vi "UIMessage1.vi"(4 "User Parameter":T1, 5 "Event Data":cluster{"uiMsg":refnum<k7>, "cancel":bool}, 6 "Control Ref":refnum<k7>, 7 "Event Common Data":T2) -> (1 "Event Data Out":cluster{"cancel":bool})   [LabVIEW 2018]
uses:
  <vilib>/Utility/miscctls.llb/LVRowAndColumnUnsignedTypeDef.ctl
  <vilib>/Utility/miscctls.llb/LVRowAndColumnTypeDef.ctl
  <vilib>/Utility/file.llb/Write Delimited Spreadsheet (string).vi
panel:
  in  "error in (no error)":errorcluster
  out "reference out":refnum<vi>
  out "error out":errorcluster
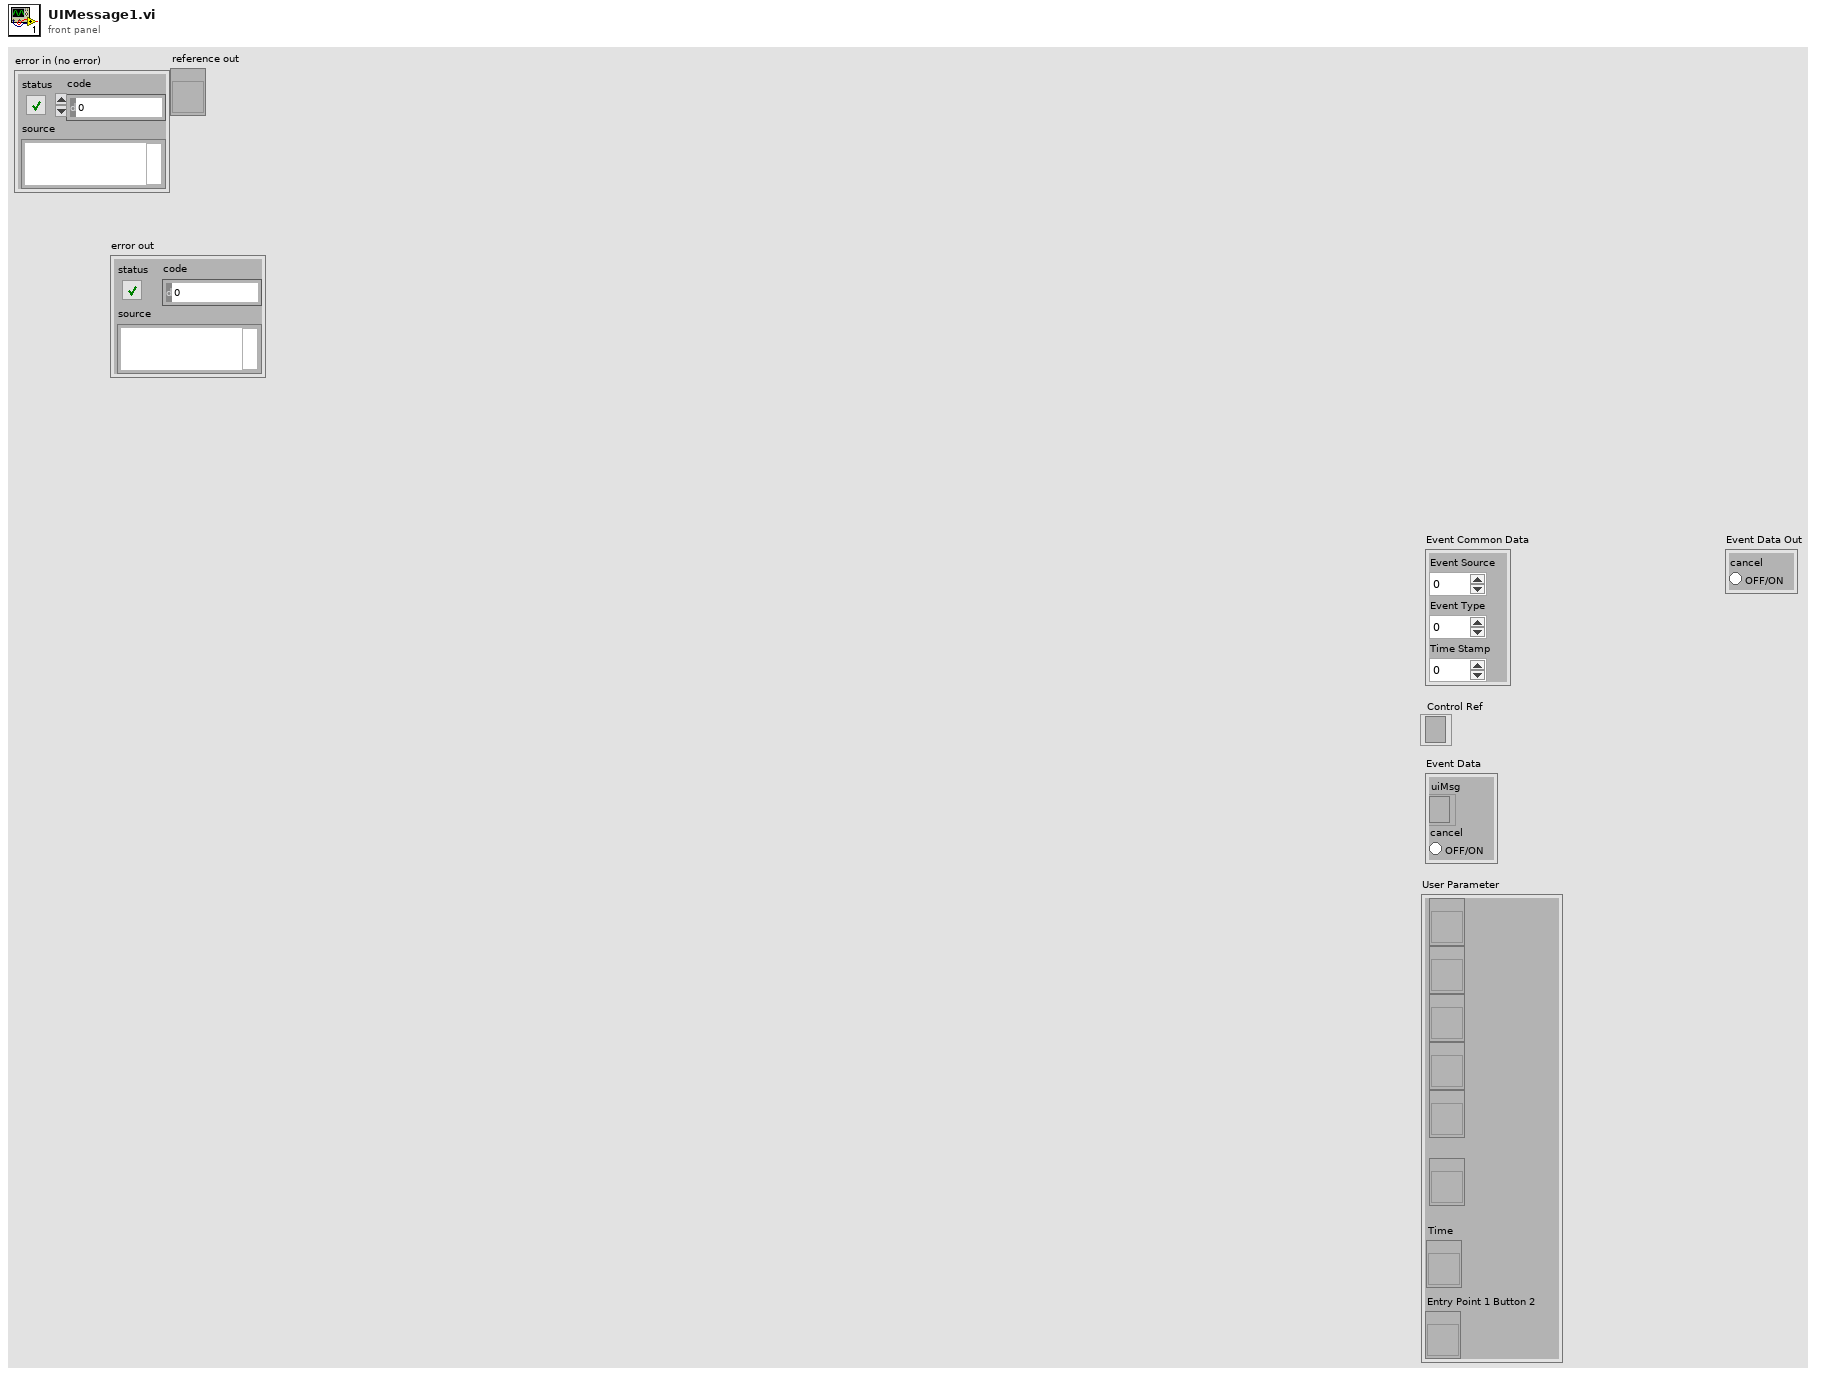
[diagram p1: front panel]
types:
  T1 = cluster{refnum<vi>, refnum<vi>, refnum<vi>, refnum<vi>, refnum<vi>, refnum<vi>, "Time":refnum<vi>, "Entry Point 1 Button 2":refnum<vi>}
  T2 = cluster{"Event Source":i32, "Event Type":u32, "Time Stamp":u32}
  T3 = typedef "LVRowAndColumnUnsignedTypeDef.ctl" = cluster{"Row":u32, "Column":u32}
  T4 = enum8{"Enabled", "Disabled", "Disabled and Grayed Out"}
  T5 = typedef "LVRowAndColumnTypeDef.ctl" = cluster{"Row":i32, "Column":i32}
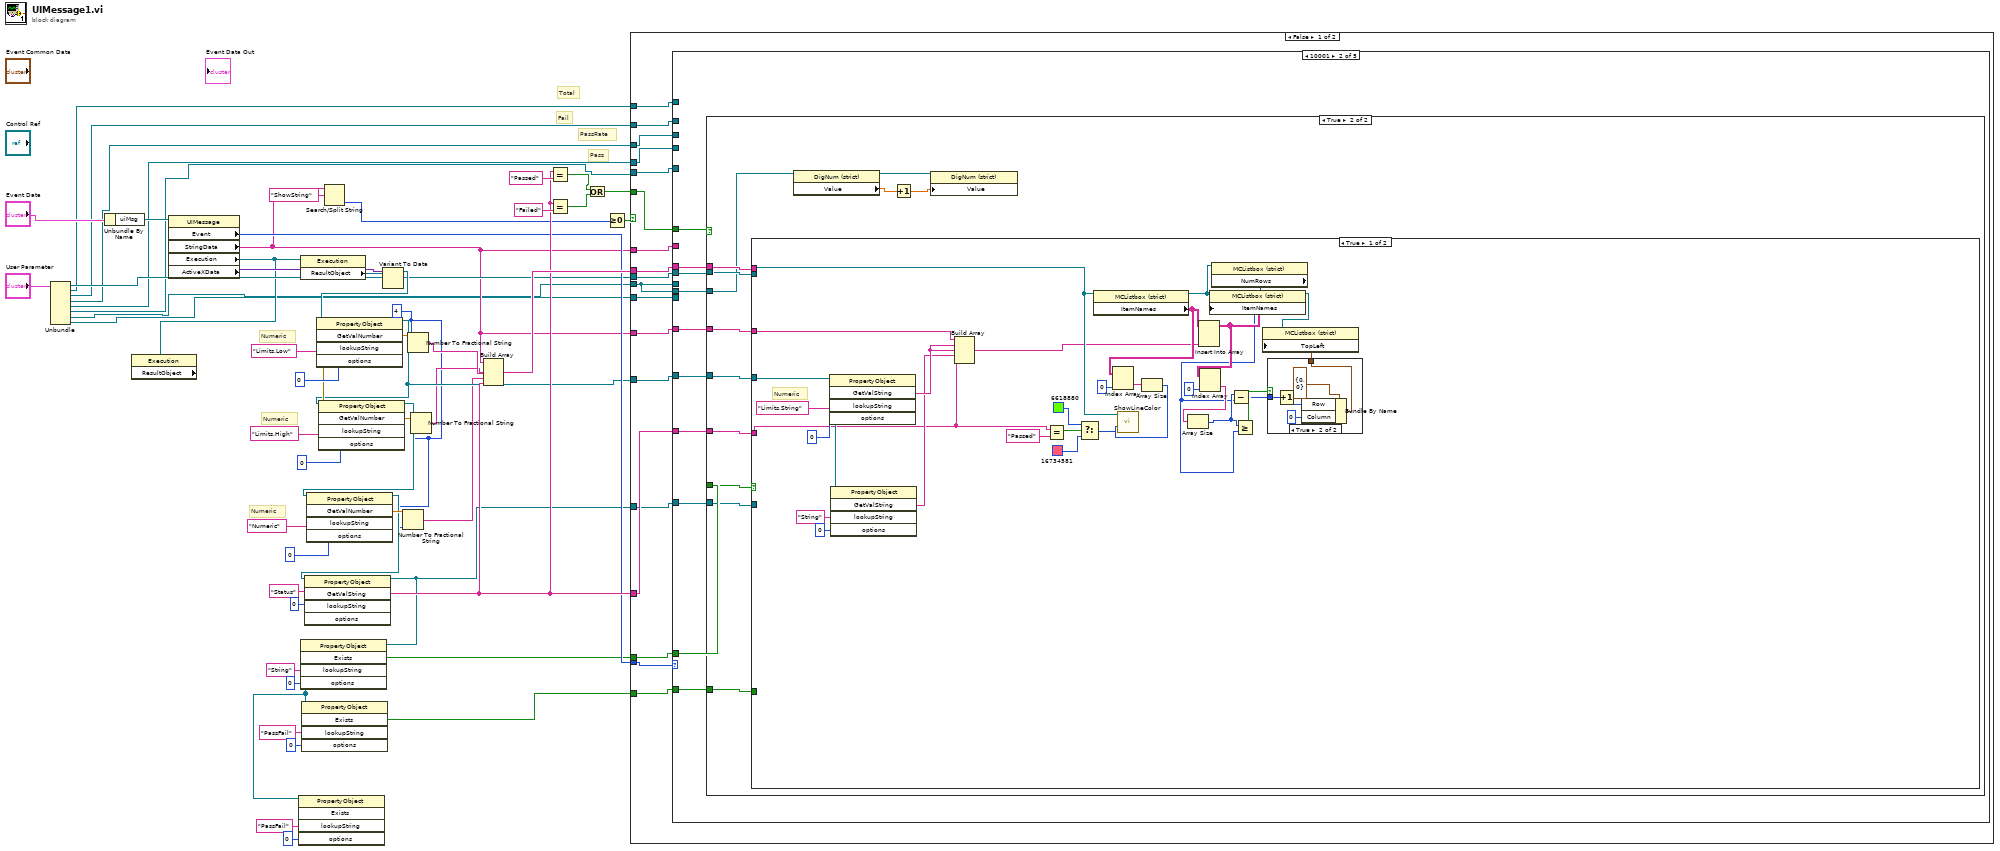
[diagram p0: block diagram]
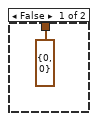
[diagram p4: hidden frame]
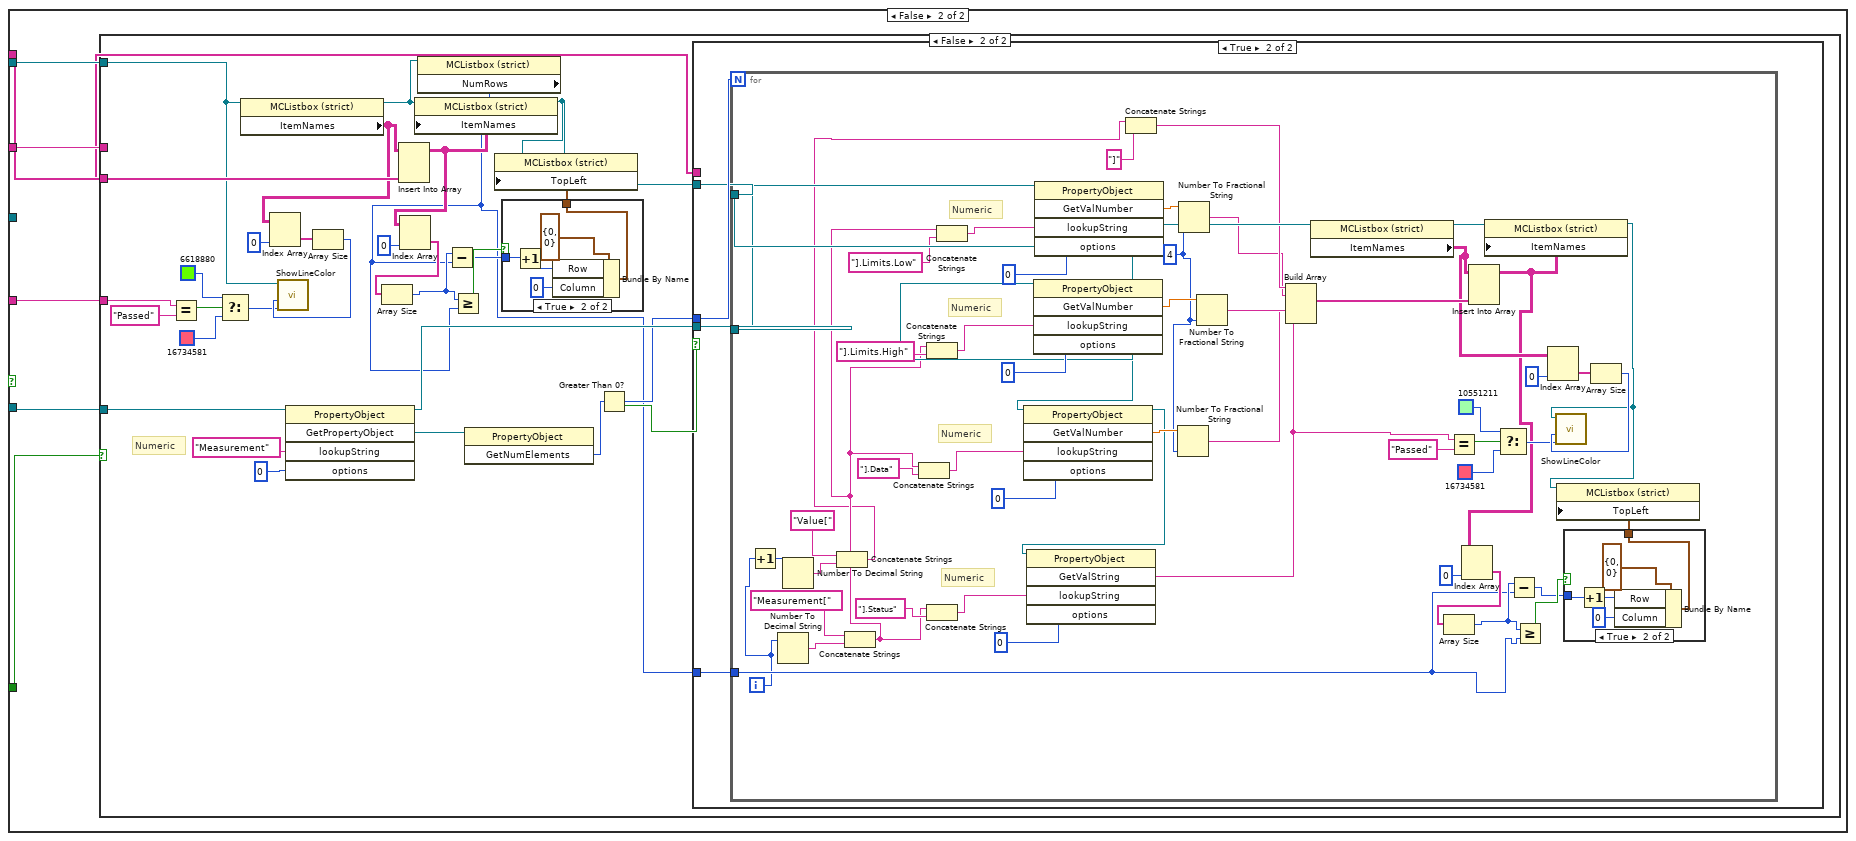
[diagram p5: hidden frame]
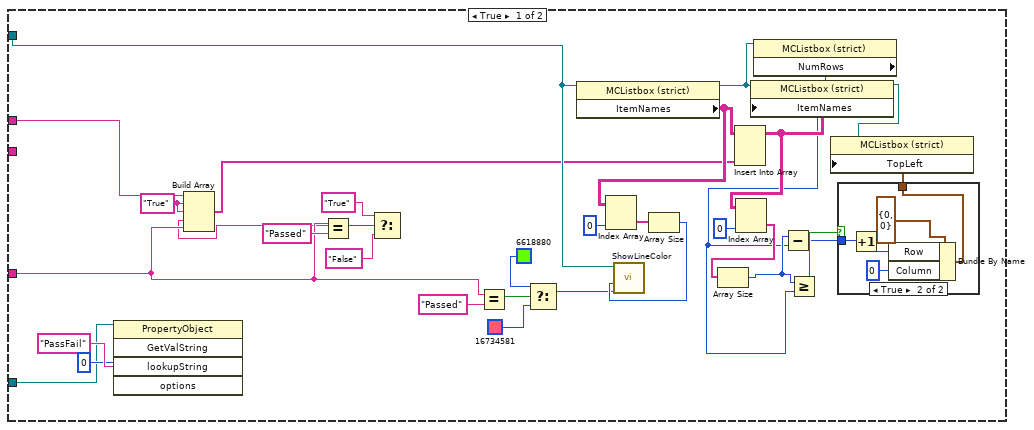
[diagram p6: hidden frame]
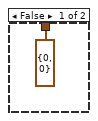
[diagram p7: hidden frame]
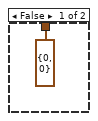
[diagram p8: hidden frame]
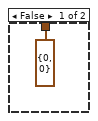
[diagram p10: hidden frame]
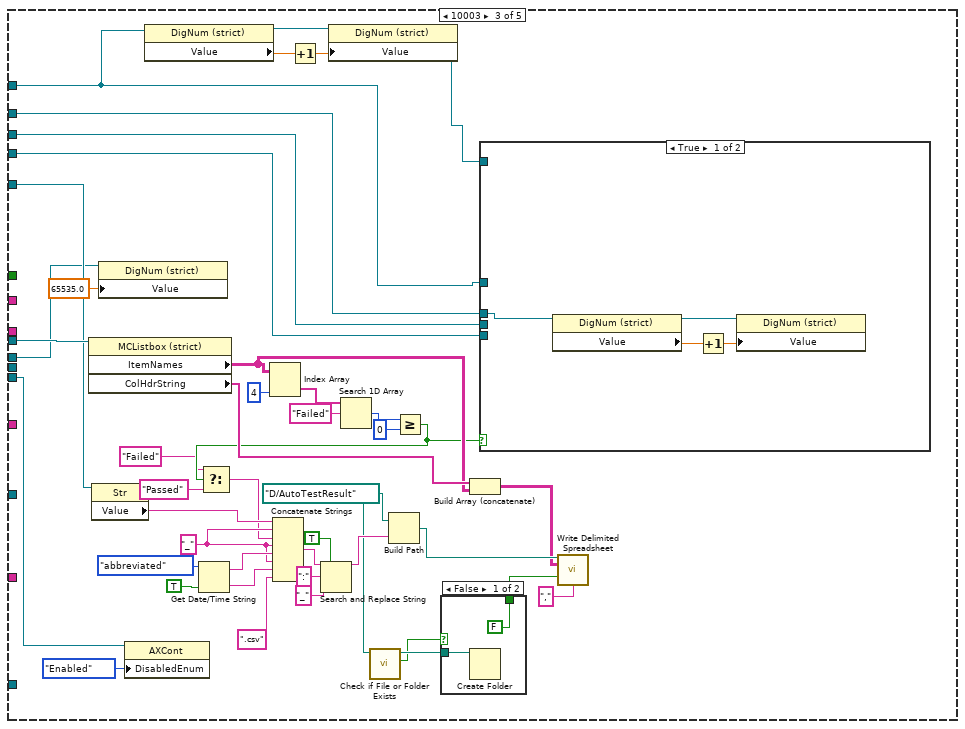
[diagram p11: hidden frame]
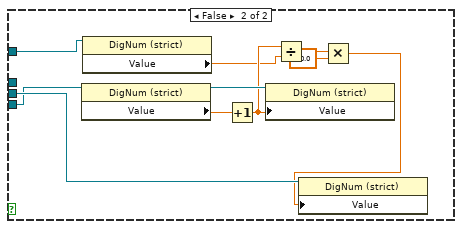
[diagram p13: hidden frame]
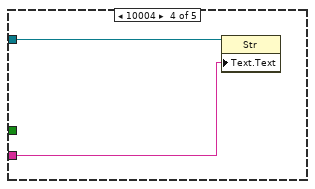
[diagram p14: hidden frame]
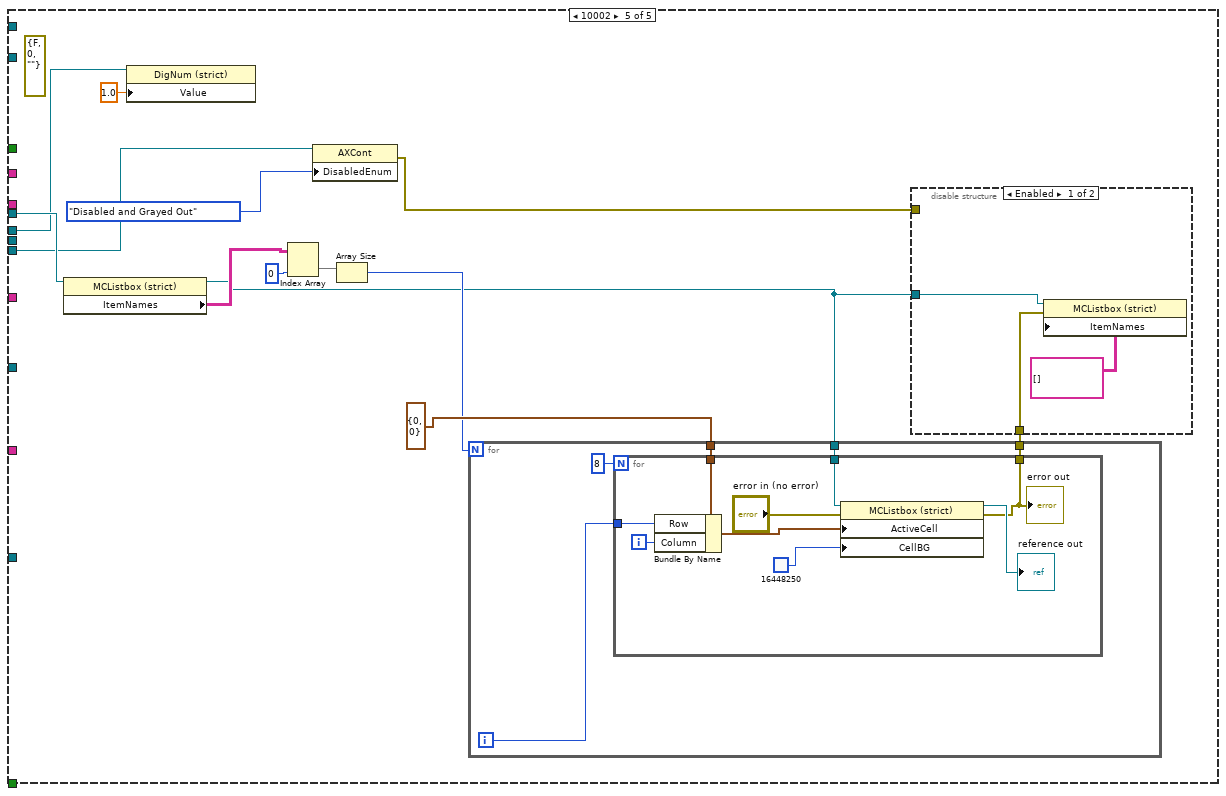
[diagram p15: hidden frame]
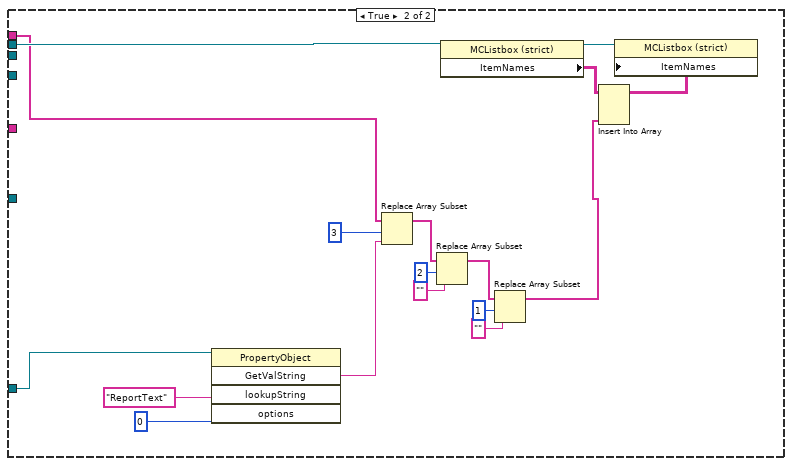
[diagram p17: hidden frame]
diagram:
  w12 = i16 4 ("precision (6)")
  # "Pass"
  # "PassRate"
  # "Fail"
  # "Total"
  # "Numeric"
  # "Numeric"
  # "Numeric"
  n1 = Unbundle("User Parameter") -> (w29:refnum<vi>, w24:refnum<vi>, w27:refnum<vi>, w26:refnum<vi>, w25:refnum<vi>, w4:refnum<vi>, "Time"=w1:refnum<vi>, "Entry Point 1 Button 2"=w2:refnum<vi>)
  n2 = Unbundle By Name("Event Data") -> ("uiMsg"=w56:refnum<k7>)
  n3 = property class="UIMessage"(reference=w56) -> ("Event"=w32:i32, "StringData"=w3:string, "Execution"=w8:refnum<k7>, "ActiveXData"=w55:variant)  [unwired: 1 in, 2 out]
  n4 = property class="Execution" props=["ResultObject"](reference=w8) -> ()  [unwired: 1 in, 3 out]
  n5 = property class="Execution"(reference=w8) -> ("ResultObject"=w52:refnum<k7>)  [unwired: 1 in, 2 out]
  n6 = Search/Split String(string=w3, search string/char (-)="ShowString") -> (offset of match=w6:i32)  [unwired: 1 in, 2 out]
  n7 = Variant To Data(type=w52, Variant=w55) -> (data=w40:refnum<k7>)  [unwired: 1 in, 1 out]
  n8 = invoke class="PropertyObject" method="GetValNumber"(reference=w40, "lookupString"="Limits.Low", "options"=0) -> (reference out=w19:refnum<k7>, error out=w42:errorcluster, "GetValNumber"=w46:dbl)  [unwired: 2 in, 2 out]
  n9 = invoke class="PropertyObject" method="GetValNumber"(reference=w19, error in=w42, "lookupString"="Limits.High", "options"=0) -> (reference out=w39:refnum<k7>, "GetValNumber"=w45:dbl)  [unwired: 1 in, 3 out]
  n10 = invoke class="PropertyObject" method="GetValNumber"(reference=w39, "lookupString"="Numeric", "options"=0) -> (reference out=w38:refnum<k7>, "GetValNumber"=w49:dbl)  [unwired: 2 in, 3 out]
  n11 = invoke class="PropertyObject" method="GetValString"(reference=w38, "lookupString"="Status", "options"=0) -> (reference out=w23:refnum<k7>, "GetValString"=w33:string)  [unwired: 2 in, 3 out]
  n12 = invoke class="PropertyObject" method="Exists"(reference=w23, "lookupString"="String", "options"=0) -> (reference out=w9:refnum<k7>, "Exists"=w20:bool)  [unwired: 2 in, 3 out]
  n13 = invoke class="PropertyObject" method="Exists"(reference=w9, "lookupString"="PassFail", "options"=0) -> ()  [unwired: 2 in, 5 out]
  n14 = invoke class="PropertyObject" method="Exists"(reference=w9, "lookupString"="PassFail", "options"=0) -> ("Exists"=w16:bool)  [unwired: 2 in, 4 out]
  n15 = Number To Fractional String(number=w49, precision (6)=w12) -> (F-format string=w13:string)  [unwired: 2 in]
  n16 = Number To Fractional String(number=w46, precision (6)=w12) -> (F-format string=w15:string)  [unwired: 2 in]
  n17 = Number To Fractional String(number=w45, precision (6)=w12) -> (F-format string=w14:string)  [unwired: 2 in]
  n18 = Build Array(w3, w15, w14, w13, w33) -> (w41:string[])
  n19 = Equal?(x=w33, y="Passed") -> (x = y?=w35:bool)
  n20 = Equal?(x=w33, y="Failed") -> (x = y?=w34:bool)
  n21 = Or(x=w35, y=w34) -> (x .or. y?=w31:bool)
  n22 = Greater Or Equal To 0?(x=w6) -> (x >= 0?=w5:bool)
  n23 = case shown="False" w5 {
    tunnel: w41 -> [w74 w379]
    tunnel: w33 -> [w73 _]
    tunnel: w32 -> [w72 _]
    tunnel: w31 -> [w71 _]
    tunnel: w29 -> [w70 w383]
    tunnel: w27 -> [w69 _]
    tunnel: w26 -> [w68 _]
    tunnel: w25 -> [w67 _]
    tunnel: w24 -> [w66 _]
    tunnel: w23 -> [w65 w380]
    tunnel: w20 -> [w64 _]
    tunnel: w19 -> [w63 _]
    tunnel: w16 -> [w62 _]
    tunnel: w3 -> [w61 _]
    tunnel: w4 -> [w60 _]
    tunnel: w3 -> [w59 _]
    tunnel: w2 -> [w58 _]
    tunnel: w1 -> [w57 _]
    frame False {
      n24 = case shown="10001" w72 {
        tunnel: w74 -> [_ w84 _ _ _]
        tunnel: w70 -> [_ w83 w321 _ w348]
        tunnel: w71 -> [_ w82 _ _ _]
        tunnel: w65 -> [_ w81 _ _ _]
        tunnel: w73 -> [_ w80 _ _ _]
        tunnel: w66 -> [_ _ w310 _ _]
        tunnel: w69 -> [_ _ w315 _ _]
        tunnel: w68 -> [_ _ w313 _ _]
        tunnel: w67 -> [_ _ w314 _ _]
        tunnel: w64 -> [_ w79 _ _ _]
        tunnel: w61 -> [_ w78 _ _ _]
        tunnel: w63 -> [_ w77 _ _ _]
        tunnel: w62 -> [_ w76 _ _ _]
        tunnel: w60 -> [_ _ w307 w339 _]
        tunnel: w59 -> [_ _ _ w338 _]
        tunnel: w58 -> [_ _ w281 _ w344]
        tunnel: w57 -> [_ _ w279 _ w340]
        tunnel: w57 -> [_ w75 _ _ _]
        frame 0, Default {
        }
        frame 10001 {
          n25 = case shown="True" w82 {
            tunnel: w84 -> [_ w96]
            tunnel: w83 -> [_ w94]
            tunnel: w81 -> [_ w95]
            tunnel: w80 -> [_ w93]
            tunnel: w79 -> [_ w92]
            tunnel: w78 -> [_ w91]
            tunnel: w77 -> [_ w90]
            tunnel: w76 -> [_ w89]
            tunnel: w75 -> [_ w86]
            frame False {
            }
            frame True {
              n26 = case shown="True" w92 {
                tunnel: w96 -> [_ w139]
                tunnel: w95 -> [_ w138]
                tunnel: w94 -> [w127 w137]
                tunnel: w93 -> [w97 w136]
                tunnel: w91 -> [w106 w134]
                tunnel: w90 -> [w104 _]
                tunnel: w89 -> [_ w135]
                frame True {
                  # "Numeric"
                  n27 = invoke class="PropertyObject" method="GetValString"(reference=w104, "lookupString"="Limits.String", "options"=0) -> (reference out=w99:refnum<k7>, "GetValString"=w102:string)  [unwired: 2 in, 3 out]
                  n28 = invoke class="PropertyObject" method="GetValString"(reference=w99, "lookupString"="String", "options"=0) -> ("GetValString"=w98:string)  [unwired: 2 in, 4 out]
                  n29 = Build Array(w106, w102, w102, w98, w97) -> (w107:string[])
                  n30 = Equal?(x=w97, y="Passed") -> (x = y?=w121:bool)
                  n31 = Select(t=u32 6618880, s=w121, f=u32 16734581) -> (s? t:f=w118:u32)
                  n32 = property on="Property Node" class="MCListbox (strict)"(reference=w127) -> (reference out=w109:refnum<vi>, "ItemNames"=w126:string[][])  [unwired: 1 in, 1 out]
                  n33 = Index Array(array=w126, index (col)=0 ("disabled index (col)")) -> (element=w124:string[])  [unwired: 1 in]
                  n34 = Array Size(array=w124) -> (size(s)=w123:i32)
                  n35 = call "ShowLineColor.vi"("ColorIn"=w118, "TestingIndex"=w123, "MulticolumnListbox in"=w127) -> ()  [unwired: 9 in]
                  n36 = Insert Into Array(array=w126, new element=w107) -> (w116:string[][])  [unwired: 2 in]
                  n37 = Index Array(array=w116, index (col)=0 ("disabled index (col)")) -> (element=w114:string[])  [unwired: 1 in]
                  n38 = Array Size(array=w114) -> (size(s)=w112:i32)
                  n39 = property on="Property Node" class="MCListbox (strict)"(reference=w109, "ItemNames"=w116) -> (reference out=w117:refnum<vi>)  [unwired: 1 in, 1 out]
                  n40 = property on="Property Node" class="MCListbox (strict)"(reference=w109) -> ("NumRows"=w108:u32)  [unwired: 1 in, 2 out]
                  n41 = Subtract(x=w112, y=w108) -> (x-y=w110:u32)
                  n42 = Greater Or Equal?(x=w112, y=w108) -> (x >= y?=w113:bool)
                  n43 = case shown="True" w113 {
                    tunnel: [T3 {"Row"=0, "Column"=0} ("Top Left Visible Cell") w131] -> w111
                    tunnel: w110 -> [_ w130]
                    frame False {
                    }
                    frame True {
                      n44 = Increment(x=w130) -> (x+1=w129:u32)
                      n45 = Bundle By Name(cluster=T3 {"Row"=0, "Column"=0} ("Top Left Visible Cell"), "Row"=w129, "Column"=u32 0) -> (w131:T3)
                    }
                  }
                  n46 = property class="MCListbox (strict)"(reference=w117, "TopLeft"=w111) -> ()  [unwired: 1 in, 2 out]
                }
                frame False {
                  n47 = case shown="False" w135 {
                    tunnel: w139 -> [_ w205]
                    tunnel: w138 -> [w146 w201]
                    tunnel: w137 -> [w171 w198]
                    tunnel: w136 -> [w143 w189]
                    tunnel: w134 -> [w151 _]
                    frame True {
                      w150 = "True" ("element")
                      n48 = invoke class="PropertyObject" method="GetValString"(reference=w146, "lookupString"="PassFail", "options"=0) -> ()  [unwired: 2 in, 5 out]
                      n49 = Equal?(x=w143, y="Passed") -> (x = y?=w145:bool)
                      n50 = Select(t="True" ("y"), s=w145, f="False" ("y")) -> (s? t:f=w140:string)
                      n51 = Build Array(w151, w150, w150, w140, w143) -> (w147:string[])
                      n52 = Equal?(x=w143, y="Passed") -> (x = y?=w165:bool)
                      n53 = Select(t=u32 6618880, s=w165, f=u32 16734581) -> (s? t:f=w162:u32)
                      n54 = property on="Property Node" class="MCListbox (strict)"(reference=w171) -> (reference out=w153:refnum<vi>, "ItemNames"=w170:string[][])  [unwired: 1 in, 1 out]
                      n55 = Index Array(array=w170, index (col)=0 ("disabled index (col)")) -> (element=w168:string[])  [unwired: 1 in]
                      n56 = Array Size(array=w168) -> (size(s)=w167:i32)
                      n57 = call "ShowLineColor.vi"("ColorIn"=w162, "TestingIndex"=w167, "MulticolumnListbox in"=w171) -> ()  [unwired: 9 in]
                      n58 = Insert Into Array(array=w170, new element=w147) -> (w160:string[][])  [unwired: 2 in]
                      n59 = Index Array(array=w160, index (col)=0 ("disabled index (col)")) -> (element=w158:string[])  [unwired: 1 in]
                      n60 = Array Size(array=w158) -> (size(s)=w156:i32)
                      n61 = property on="Property Node" class="MCListbox (strict)"(reference=w153, "ItemNames"=w160) -> (reference out=w161:refnum<vi>)  [unwired: 1 in, 1 out]
                      n62 = property on="Property Node" class="MCListbox (strict)"(reference=w153) -> ("NumRows"=w152:u32)  [unwired: 1 in, 2 out]
                      n63 = Subtract(x=w156, y=w152) -> (x-y=w154:u32)
                      n64 = Greater Or Equal?(x=w156, y=w152) -> (x >= y?=w157:bool)
                      n65 = case shown="True" w157 {
                        tunnel: [T3 {"Row"=0, "Column"=0} ("Top Left Visible Cell") w175] -> w155
                        tunnel: w154 -> [_ w174]
                        frame False {
                        }
                        frame True {
                          n66 = Increment(x=w174) -> (x+1=w173:u32)
                          n67 = Bundle By Name(cluster=T3 {"Row"=0, "Column"=0} ("Top Left Visible Cell"), "Row"=w173, "Column"=u32 0) -> (w175:T3)
                        }
                      }
                      n68 = property class="MCListbox (strict)"(reference=w161, "TopLeft"=w155) -> ()  [unwired: 1 in, 2 out]
                    }
                    frame False {
                      # "Numeric"
                      n69 = Equal?(x=w189, y="Passed") -> (x = y?=w192:bool)
                      n70 = Select(t=u32 6618880, s=w192, f=u32 16734581) -> (s? t:f=w188:u32)
                      n71 = property on="Property Node" class="MCListbox (strict)"(reference=w198) -> (reference out=w179:refnum<vi>, "ItemNames"=w197:string[][])  [unwired: 1 in, 1 out]
                      n72 = Index Array(array=w197, index (col)=0 ("disabled index (col)")) -> (element=w195:string[])  [unwired: 1 in]
                      n73 = invoke class="PropertyObject" method="GetPropertyObject"(reference=w201, "lookupString"="Measurement", "options"=0) -> (reference out=w200:refnum<k7>, "GetPropertyObject"=w204:refnum<k7>)  [unwired: 2 in, 3 out]
                      n74 = Array Size(array=w195) -> (size(s)=w194:i32)
                      n75 = call "ShowLineColor.vi"("ColorIn"=w188, "TestingIndex"=w194, "MulticolumnListbox in"=w198) -> ()  [unwired: 9 in]
                      n76 = Insert Into Array(array=w197, new element=w205) -> (w186:string[][])  [unwired: 2 in]
                      n77 = Index Array(array=w186, index (col)=0 ("disabled index (col)")) -> (element=w184:string[])  [unwired: 1 in]
                      n78 = Array Size(array=w184) -> (size(s)=w182:i32)
                      n79 = property on="Property Node" class="MCListbox (strict)"(reference=w179, "ItemNames"=w186) -> (reference out=w187:refnum<vi>)  [unwired: 1 in, 1 out]
                      n80 = property on="Property Node" class="MCListbox (strict)"(reference=w179) -> ("NumRows"=w178:u32)  [unwired: 1 in, 2 out]
                      n81 = Subtract(x=w182, y=w178) -> (x-y=w180:u32)
                      n82 = Greater Or Equal?(x=w182, y=w178) -> (x >= y?=w183:bool)
                      n83 = invoke class="PropertyObject" method="GetNumElements"(reference=w204) -> ("GetNumElements"=w199:i32)  [unwired: 2 in, 2 out]
                      n84 = case shown="True" w183 {
                        tunnel: [T3 {"Row"=0, "Column"=0} ("Top Left Visible Cell") w210] -> w181
                        tunnel: w180 -> [_ w209]
                        frame False {
                        }
                        frame True {
                          n85 = Increment(x=w209) -> (x+1=w208:u32)
                          n86 = Bundle By Name(cluster=T3 {"Row"=0, "Column"=0} ("Top Left Visible Cell"), "Row"=w208, "Column"=u32 0) -> (w210:T3)
                        }
                      }
                      n87 = property class="MCListbox (strict)"(reference=w187, "TopLeft"=w181) -> ()  [unwired: 1 in, 2 out]
                      n88 = Greater Than 0?(x=w199) -> (x > 0?=w206:bool)
                      n89 = case shown="True" w206 {
                        tunnel: w199 -> [_ w216]
                        tunnel: w200 -> [_ w215]
                        tunnel: w205 -> [_ _]
                        tunnel: w187 -> [_ w214]
                        tunnel: w178 -> [_ w213]
                        frame False {
                        }
                        frame True {
                          n90 = for {
                            N: w216 -> [_]
                            tunnel: w215 -> [w261]
                            tunnel: w214 -> [w271]
                            tunnel: w213 -> [w228]
                            i -> [w225]
                            w217 = i16 4 ("precision (6)")
                            # "Numeric"
                            # "Numeric"
                            # "Numeric"
                            # "Numeric"
                            n91 = Increment(x=w225) -> (x+1=w224:i32)
                            n92 = Number To Decimal String(number=w225) -> (decimal integer string=w258:string)  [unwired: 1 in]
                            n93 = Number To Decimal String(number=w224) -> (decimal integer string=w223:string)  [unwired: 1 in]
                            n94 = Concatenate Strings("Value[" ("string"), w223) -> (w222:string)
                            n95 = Concatenate Strings("Measurement[" ("string"), w258) -> (w227:string)
                            n96 = Concatenate Strings(w227, "].Data" ("lookupString")) -> (w251:string)
                            n97 = Concatenate Strings(w227, "].Limits.High" ("lookupString")) -> (w253:string)
                            n98 = Concatenate Strings(w227, "].Status" ("lookupString")) -> (w249:string)
                            n99 = Concatenate Strings(w227, "].Limits.Low" ("lookupString")) -> (w255:string)
                            n100 = invoke class="PropertyObject" method="GetValNumber"(reference=w261, "lookupString"=w255, "options"=0) -> (reference out=w266:refnum<k7>, "GetValNumber"=w268:dbl)  [unwired: 2 in, 3 out]
                            n101 = invoke class="PropertyObject" method="GetValNumber"(reference=w266, "lookupString"=w253, "options"=0) -> (reference out=w262:refnum<k7>, "GetValNumber"=w265:dbl)  [unwired: 2 in, 3 out]
                            n102 = invoke class="PropertyObject" method="GetValNumber"(reference=w262, "lookupString"=w251, "options"=0) -> (reference out=w259:refnum<k7>, "GetValNumber"=w264:dbl)  [unwired: 2 in, 3 out]
                            n103 = invoke class="PropertyObject" method="GetValString"(reference=w259, "lookupString"=w249, "options"=0) -> ("GetValString"=w238:string)  [unwired: 2 in, 4 out]
                            n104 = Concatenate Strings(w222, "]" ("string")) -> (w221:string)
                            n105 = Number To Fractional String(number=w264, precision (6)=w217) -> (F-format string=w218:string)  [unwired: 2 in]
                            n106 = Number To Fractional String(number=w268, precision (6)=w217) -> (F-format string=w220:string)  [unwired: 2 in]
                            n107 = Number To Fractional String(number=w265, precision (6)=w217) -> (F-format string=w219:string)  [unwired: 2 in]
                            n108 = Build Array(w221, w220, w219, w218, w238) -> (w270:string[])
                            n109 = property on="Property Node" class="MCListbox (strict)"(reference=w271) -> (reference out=w248:refnum<vi>, "ItemNames"=w239:string[][])  [unwired: 1 in, 1 out]
                            n110 = Equal?(x=w238, y="Passed") -> (x = y?=w244:bool)
                            n111 = Insert Into Array(array=w239, new element=w270) -> (w232:string[][])  [unwired: 2 in]
                            n112 = Index Array(array=w232, index (col)=0 ("disabled index (col)")) -> (element=w234:string[])  [unwired: 1 in]
                            n113 = Array Size(array=w234) -> (size(s)=w235:i32)
                            n114 = property on="Property Node" class="MCListbox (strict)"(reference=w248, "ItemNames"=w232) -> (reference out=w230:refnum<vi>)  [unwired: 1 in, 1 out]
                            n115 = Select(t=u32 10551211, s=w244, f=u32 16734581) -> (s? t:f=w237:u32)
                            n116 = Subtract(x=w235, y=w228) -> (x-y=w229:u32)
                            n117 = Greater Or Equal?(x=w235, y=w228) -> (x >= y?=w231:bool)
                            n118 = Index Array(array=w239, index (col)=0 ("disabled index (col)")) -> (element=w241:string[])  [unwired: 1 in]
                            n119 = case shown="True" w231 {
                              tunnel: [T3 {"Row"=0, "Column"=0} ("Top Left Visible Cell") w275] -> w236
                              tunnel: w229 -> [_ w274]
                              frame False {
                              }
                              frame True {
                                n120 = Increment(x=w274) -> (x+1=w273:u32)
                                n121 = Bundle By Name(cluster=T3 {"Row"=0, "Column"=0} ("Top Left Visible Cell"), "Row"=w273, "Column"=u32 0) -> (w275:T3)
                              }
                            }
                            n122 = property class="MCListbox (strict)"(reference=w230, "TopLeft"=w236) -> ()  [unwired: 1 in, 2 out]
                            n123 = Array Size(array=w241) -> (size(s)=w242:i32)
                            n124 = call "ShowLineColor.vi"("ColorIn"=w237, "TestingIndex"=w242, "MulticolumnListbox in"=w230) -> ()  [unwired: 9 in]
                          }
                        }
                      }
                    }
                  }
                }
              }
              n125 = property class="DigNum (strict)"(reference=w86) -> (reference out=w85:refnum<vi>, "Value"=w88:dbl)  [unwired: 1 in, 1 out]
              n126 = Increment(x=w88) -> (x+1=w87:dbl)
              n127 = property class="DigNum (strict)"(reference=w85, "Value"=w87) -> ()  [unwired: 1 in, 2 out]
            }
          }
        }
        frame 10003 {
          w286 = "_" ("string")
          w290 = path "D:/AutoTestResult" ("file path (dialog if empty)")
          n128 = property class="MCListbox (strict)"(reference=w321) -> ("ItemNames"=w299:string[][], "ColHdrString"=w300:string[])  [unwired: 1 in, 2 out]
          n129 = property class="Str"(reference=w307) -> ("Value"=w306:string)  [unwired: 1 in, 2 out]
          n130 = property class="DigNum (strict)"(reference=w279, "Value"=65535.0) -> ()  [unwired: 1 in, 2 out]
          n131 = property class="AXCont"(reference=w281, "DisabledEnum"=T4."Enabled" ("Disabled")) -> ()  [unwired: 1 in, 2 out]
          n132 = property class="DigNum (strict)"(reference=w310) -> (reference out=w308:refnum<vi>, "Value"=w312:dbl)  [unwired: 1 in, 1 out]
          n133 = Get Date/Time String(date format (0)=enum16{"short", "long", "abbreviated"}."abbreviated" ("日期格式(0)"), want seconds? (F)=TRUE ("需要秒？(F)")) -> (date string=w303:string, time string=w302:string)  [unwired: 1 in]
          n134 = Index Array(array=w299, index (col)=4 ("disabled index (col)")) -> (element=w319:string[])  [unwired: 1 in]
          n135 = Increment(x=w312) -> (x+1=w311:dbl)
          n136 = property class="DigNum (strict)"(reference=w308, "Value"=w311) -> (reference out=w309:refnum<vi>)  [unwired: 1 in, 1 out]
          n137 = Search 1D Array(1D array=w319, element="Failed") -> (index of element=w317:i32)  [unwired: 1 in]
          n138 = call <vilib>:"Check if File or Folder Exists.vi"("path"=w290) -> ("file or folder exists?"=w288:bool, "dup path"=w289:path)  [unwired: 8 in, 1 out]
          n139 = Greater Or Equal?(x=w317, y=0) -> (x >= y?=w285:bool)
          n140 = Select(t="Failed" ("string"), s=w285, f="Passed" ("y")) -> (s? t:f=w282:string)
          n141 = Concatenate Strings(w306, w286, w282, w286, w303, w286, w302, ".csv" ("string")) -> (w295:string)
          n142 = Search and Replace String(replace all?=TRUE ("replace all? (F)"), input string=w295, search string=":", replace string="_" ("replace string (\"\")")) -> (result string=w292:string)  [unwired: 4 in, 3 out]
          n143 = Build Path(base path=w290, name or relative path=w292) -> (appended path=w301:path)
          n144 = case shown="False" w288 {
            tunnel: w289 -> [w323 _]
            tunnel: [FALSE ("append to file? (new file:F)") _] -> w287
            frame False {
              n145 = Create Folder(path (use dialog)=w323) -> ()  [unwired: 2 in, 3 out]
            }
            frame True {
            }
          }
          n146 = Build Array (concatenate)(w300, w299) -> (w298:string[][])
          n147 = case shown="True" w285 {
            tunnel: w315 -> [w324 _]
            tunnel: w314 -> [_ w328]
            tunnel: w310 -> [_ w335]
            tunnel: w313 -> [_ w330]
            tunnel: w309 -> [_ _]
            frame True {
              n148 = property class="DigNum (strict)"(reference=w324) -> (reference out=w327:refnum<vi>, "Value"=w326:dbl)  [unwired: 1 in, 1 out]
              n149 = Increment(x=w326) -> (x+1=w325:dbl)
              n150 = property class="DigNum (strict)"(reference=w327, "Value"=w325) -> ()  [unwired: 1 in, 2 out]
            }
            frame False {
              n151 = property class="DigNum (strict)"(reference=w328) -> (reference out=w337:refnum<vi>, "Value"=w336:dbl)  [unwired: 1 in, 1 out]
              n152 = property class="DigNum (strict)"(reference=w335) -> ("Value"=w333:dbl)  [unwired: 1 in, 2 out]
              n153 = Increment(x=w336) -> (x+1=w334:dbl)
              n154 = property class="DigNum (strict)"(reference=w337, "Value"=w334) -> ()  [unwired: 1 in, 2 out]
              n155 = Divide(x=w334, y=w333) -> (x/y=w332:dbl)
              n156 = Multiply(x=w332, y=100.0) -> (x*y=w329:dbl)
              n157 = property class="DigNum (strict)"(reference=w330, "Value"=w329) -> ()  [unwired: 1 in, 2 out]
            }
          }
          n158 = call-poly <vilib>:"Write Delimited Spreadsheet.vi"("file path (dialog if empty)"=w301, "2D data"=w298, "append to file? (new file:F)"=w287, "delimiter (\\t)"="," ("delimiter (\\t)")) -> ()  [unwired: 10 in, 2 out]
        }
        frame 10004 {
          n159 = property class="Str"(reference=w339, "Text.Text"=w338) -> ()  [unwired: 1 in, 2 out]
        }
        frame 10002 {
          (unwired) errorcluster {"status"=FALSE, "code"=0, "source"=""} ("error in (no error)")
          n160 = property class="MCListbox (strict)"(reference=w348) -> (reference out=w346:refnum<vi>, "ItemNames"=w347:string[][])  [unwired: 1 in, 1 out]
          n161 = property class="DigNum (strict)"(reference=w340, "Value"=1.0) -> ()  [unwired: 1 in, 2 out]
          n162 = Index Array(array=w347, index (col)=0 ("disabled index (col)")) -> (element=w350:string[])  [unwired: 1 in]
          n163 = property class="AXCont"(reference=w344, "DisabledEnum"=T4."Disabled and Grayed Out" ("Disabled")) -> (error out=w342:errorcluster)  [unwired: 1 in, 1 out]
          n164 = Array Size(array=w350) -> (size(s)=w349:i32)
          n165 = for {
            N: w349 -> [_]
            tunnel: T5 {"Row"=0, "Column"=0} ("Active Cell:Active Cell") -> [w360]
            tunnel: [w359] -> w345
            tunnel: w346 -> [w356]
            i -> [w357]
            n166 = for {
              N: 8 -> [_]
              tunnel: w357 -> [w368]
              tunnel: w360 -> [w367]
              tunnel: [w362] -> w359
              tunnel: w356 -> [w361]
              i -> [w366]
              n167 = Bundle By Name(cluster=w367, "Row"=w368, "Column"=w366) -> (w369:T5)
              n168 = property on="Property Node" class="MCListbox (strict)"(reference=w361, error in="error in (no error)", "ActiveCell"=w369, "CellBG"=u32 16448250) -> (reference out=→"reference out":refnum<vi>, error out=w362:errorcluster)
              "error out" <- w362
            }
          }
          n169 = disable-structure shown="Enabled" {
            disable-tunnel: w346 -> [w355 _]
            disable-tunnel: w345 -> [w354 _]
            disable-tunnel: w342 -> [_ _]
            frame Enabled {
              n170 = property class="MCListbox (strict)"(reference=w355, error in=w354, "ItemNames"=string[][] [] ("Item Names")) -> ()  [unwired: 2 out]
            }
            frame Disabled {
            }
          }
        }
      }
    }
    frame True {
      n171 = invoke class="PropertyObject" method="GetValString"(reference=w380, "lookupString"="ReportText", "options"=0) -> ("GetValString"=w378:string)  [unwired: 2 in, 4 out]
      n172 = Replace Array Subset(array=w379, new element=w378, index=3) -> (w376:string[])
      n173 = Replace Array Subset(array=w376, new element="" ("new element/subarray"), index=2) -> (w371:string[])
      n174 = property on="Property Node" class="MCListbox (strict)"(reference=w383) -> (reference out=w384:refnum<vi>, "ItemNames"=w386:string[][])  [unwired: 1 in, 1 out]
      n175 = Replace Array Subset(array=w371, new element="" ("new element/subarray"), index=1) -> (w370:string[])
      n176 = Insert Into Array(array=w386, new element=w370) -> (w385:string[][])  [unwired: 2 in]
      n177 = property on="Property Node" class="MCListbox (strict)"(reference=w384, "ItemNames"=w385) -> ()  [unwired: 1 in, 2 out]
    }
  }
